vi "Gamepad Drive.vi"() -> (0 "Xbox":T1)   [LabVIEW 2014]
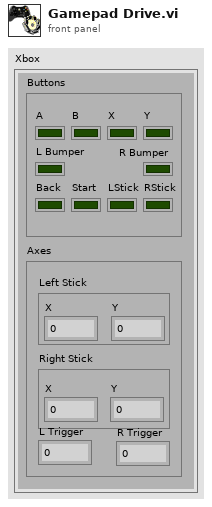
[diagram p1: front panel]
types:
  T1 = cluster{"Buttons":cluster{"A":bool, "B":bool, "X":bool, "Y":bool, "L Bumper":bool, "R Bumper":bool, "Back":bool, "Start":bool, "LStick":bool, "RStick":bool}, "Axes":cluster{"Left Stick":cluster{"X":dbl, "Y":dbl}, "Right Stick":cluster{"X":dbl, "Y":dbl}, "L Trigger":dbl, "R Trigger":dbl}}
  T2 = cluster{"Left Stick":cluster{"X":dbl, "Y":dbl}, "Right Stick":cluster{"X":dbl, "Y":dbl}, "L Trigger":dbl, "R Trigger":dbl}
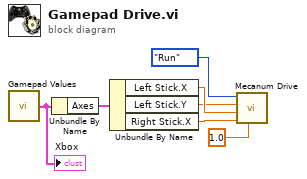
[diagram p0: block diagram]
diagram:
  n1 = call "Gamepad Values.vi"() -> ("Xbox"=w1:T1)
  "Xbox" <- w1
  n2 = Unbundle By Name(w1) -> ("Axes"=w2:T2)
  n3 = Unbundle By Name(w2) -> ("Left Stick.X"=w5:dbl, "Left Stick.Y"=w4:dbl, "Right Stick.X"=w3:dbl)
  n4 = call "Mecanum Drive.vi"("Division"=1.0, "Turn"=w3, "Strafe"=w5, "Forward/Backward"=w4, "Mode"=enum8{"Start", "Run", "Finish"}."Run") -> ()  [unwired: 7 in]
